vi "DecodeDeviceJSONList.vi"(1 "JSON":string, 5 "error in":errorcluster) -> (14 "deviceType":string, 15 "index":i32, 16 "productId":i32, 17 "serialNumber":string, 18 "isOpen":bool, 19 "error out":errorcluster)   [LabVIEW 2023, in "horiba.lvlib" / "GenericDevice.lvclass"]
doc: "Decodes the answer from the ICL into a device."
uses:
  GenericDevice.lvclass
  DecodeDevice.ctl
  221d436b-eb94-4626-8a62-798962724428.vi
  <vilib>/JDP Science/JSONtext/JSON text to Variant.vi
  <vilib>/JDP Science/JSONtext/LVClass Serializer/JSONtext LVClass Serializer.lvclass
  GenericDevice.lvclass/GenericDevice.ctl
panel:
  # "Connector Pane"
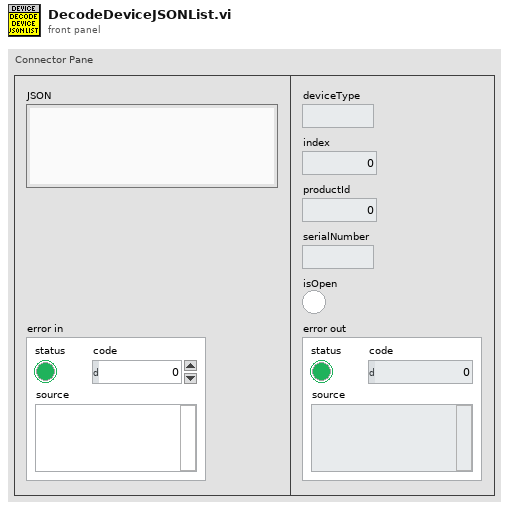
[diagram p1: front panel]
types:
  T1 = typedef "horiba.lvlib/GenericDevice.lvclass/DecodeDevice.ctl" = cluster{"deviceType":string, "index":i32, "isOpen":bool, "productId":i32, "serialNumber":string}
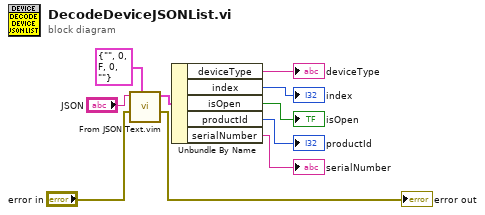
[diagram p0: block diagram]
diagram:
  n1 = call "From JSON Text.vim"("Data Type and Default Value"=T1 {"deviceType"="", "index"=0, "isOpen"=FALSE, "productId"=0, "serialNumber"=""} ("Chipsize"), "error in (no error)"="error in", "JSON"="JSON") -> ("error out"=→"error out":errorcluster, "Data out"=w10:T1)  [unwired: 7 in]
  n2 = Unbundle By Name(w10) -> ("deviceType"=→"deviceType":string, "index"=→"index":i32, "isOpen"=→"isOpen":bool, "productId"=→"productId":i32, "serialNumber"=→"serialNumber":string)
